vi "5.1.vi"() -> ()   [LabVIEW 2017]
panel:
  out "任务一":string
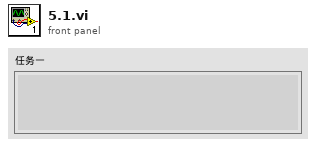
[diagram p1: front panel]
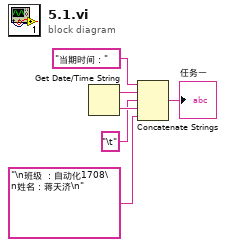
[diagram p0: block diagram]
diagram:
  n1 = Get Date/Time String() -> (date string=w4:string, time string=w3:string)  [unwired: 3 in]
  n2 = Concatenate Strings("当期时间：", w4, "\t", w3, "\n班级 ：自动化1708\n姓名：蒋天济\n") -> (→"任务一":string)
